vi "piezoEtlGetPosFromCount.vi"(4 "piezoEtlDerivativesReferences":refnum<data-value>[](array[refnum]), 5 "piezoEtlPositionsReferences":refnum<data-value>[](array[refnum]), 6 "hamamatsuFrameCounterReferences":refnum<data-value>[](array[refnum]), 7 "frameCount":u32) -> (0 "success":bool, 1 "piezoEtlDerivative":i16, 2 "piezoEtlPosition":dbl, 3 "bufferIndex":i32)   [LabVIEW 2017]
uses:
  globalDevices.vi
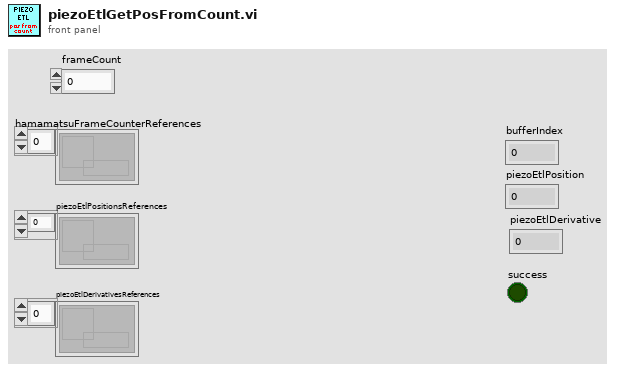
[diagram p1: front panel]
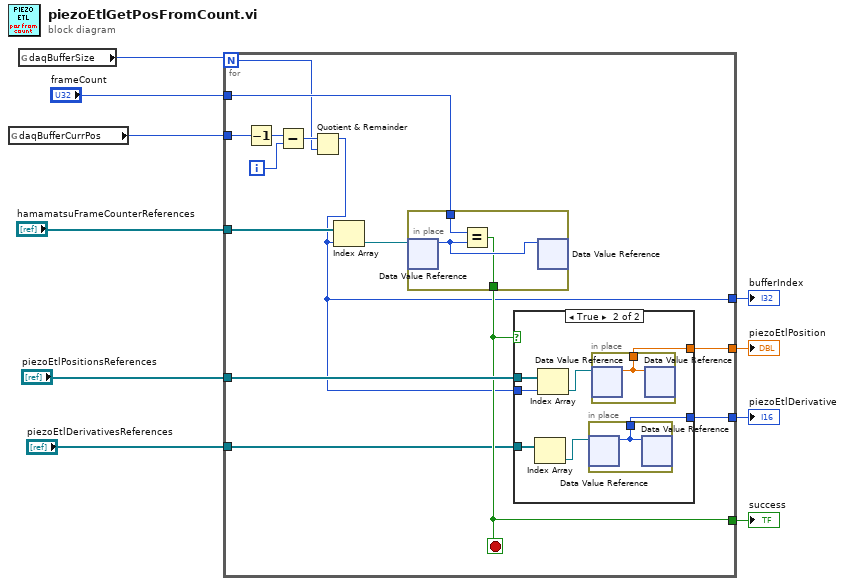
[diagram p0: block diagram]
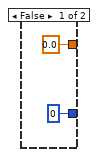
[diagram p2: hidden frame]
diagram:
  n1 = global read "globalDevices.vi" "daqBufferCurrPos"() -> (w9:i32)
  n2 = global read "globalDevices.vi" "daqBufferSize"() -> (w10:i32)
  n3 = for {
    N: w10 -> [w12]
    tunnel: w9 -> [w24]
    tunnel: "hamamatsuFrameCounterReferences" -> [w23]
    tunnel: "piezoEtlPositionsReferences" -> [w18]
    tunnel: "frameCount" -> [w19]
    tunnel: [w17] -> w1
    tunnel: [w16] -> w4
    tunnel: [w11] -> w5
    tunnel: "piezoEtlDerivativesReferences" -> [w15]
    tunnel: [w14] -> w2
    i -> [w21]
    stop <- w17 stop-if-true
    n4 = Decrement(x=w24) -> (x-1=w22:i32)
    n5 = Subtract(x=w22, y=w21) -> (x-y=w13:i32)
    n6 = Quotient & Remainder(x=w13, y=w12) -> (x-y*floor(x/y)=w11:i32)  [unwired: 1 out]
    n7 = Index Array(array=w23, index=w11) -> (element=w20:refnum<data-value>)
    n8 = in-place {
      in-place-border: w19 -> [w38]
      in-place-border: [w36] -> w17
      n9 = in-place-dvr #1(w20) -> (w37:u32)  [unwired: 1 out]
      n10 = Equal?(x=w38, y=w37) -> (x = y?=w36:bool)
      n11 = in-place-dvr #1(w37) -> ()  [unwired: 2 out]
    }
    n12 = case shown="True" w17 {
      tunnel: w18 -> [_ w33]
      tunnel: w11 -> [_ w32]
      tunnel: [0.0 w30] -> w16
      tunnel: w15 -> [_ w28]
      tunnel: [i16 0 w27] -> w14
      frame False {
      }
      frame True {
        n13 = Index Array(array=w28) -> (element=w29:refnum<data-value>)  [unwired: 1 in]
        n14 = Index Array(array=w33, index=w32) -> (element=w31:refnum<data-value>)
        n15 = in-place {
          in-place-border: [w34] -> w27
          n16 = in-place-dvr #2(w29) -> (w34:i16)  [unwired: 1 out]
          n17 = in-place-dvr #2(w34) -> ()  [unwired: 2 out]
        }
        n18 = in-place {
          in-place-border: [w35] -> w30
          n19 = in-place-dvr #3(w31) -> (w35:dbl)  [unwired: 1 out]
          n20 = in-place-dvr #3(w35) -> ()  [unwired: 2 out]
        }
      }
    }
  }
  "bufferIndex" <- w5
  "piezoEtlPosition" <- w4
  "piezoEtlDerivative" <- w2
  "success" <- w1
